vi "delay_read_points.vi"(3 "error in (no error)":errorcluster, 5 "file path (dialog if empty)":path) -> (0 "error out":errorcluster, 1 "Delay List":string[][](array[string]))   [LabVIEW 2019]
doc: "Reads in a delay list"
uses:
  <vilib>/Utility/file.llb/Read Delimited Spreadsheet (string).vi
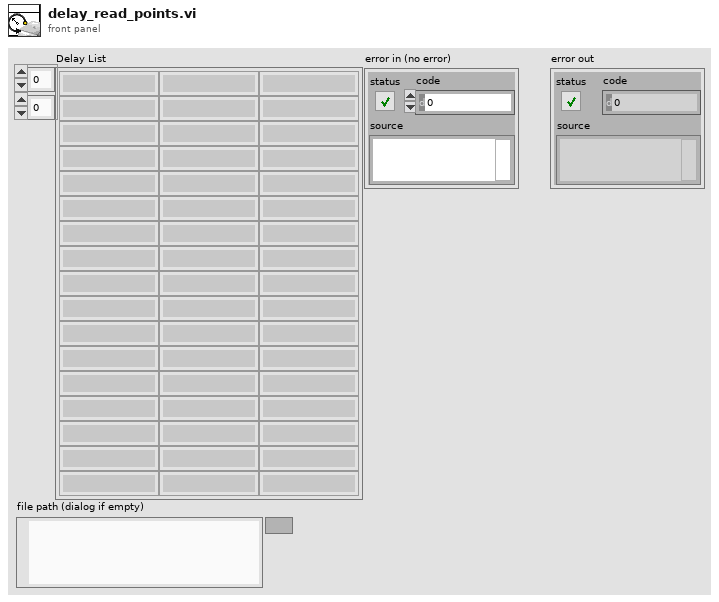
[diagram p1: front panel]
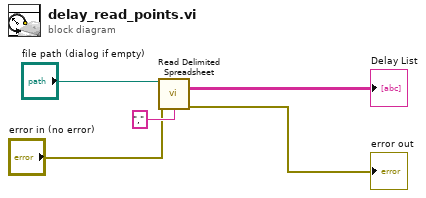
[diagram p0: block diagram]
diagram:
  n1 = call-poly <vilib>:"Read Delimited Spreadsheet.vi"("file path (dialog if empty)"="file path (dialog if empty)", "error in (no error)"="error in (no error)", "delimiter (\\t)"="," ("delimiter (\\t)")) -> ("all rows"=→"Delay List":string[][], "error out"=→"error out":errorcluster)  [unwired: 7 in, 4 out]
